vi "Read Persistent Layers.vi"(11 "Spawn in":refnum<class "Spawn.lvclass">) -> (2 "Persistent Layers":refnum<class "Actor.lvclass">[](array[class]))   [LabVIEW 2025, in "jettl.lvlib" / "Spawn.lvlib" / "Spawn.lvclass"]
uses:
  Spawn.lvclass
  Actor/Actor.lvclass
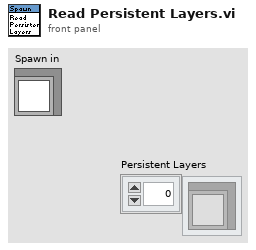
[diagram p1: front panel]
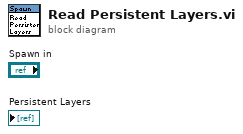
[diagram p0: block diagram]
diagram:
